vi "Wysyllanie danych do PC .vi"(5 "remote port":u16, 6 "output cluster 2":T2 {"CAN frame"."type" items=["CAN Data", "CAN Remote"]; "CAN frame"."identifier" format="%.0x"}, 7 "adres":u32, 8 "error in (no error)":errorcluster, 11 "UDP Network Connection in":refnum<k16>) -> (0 "error out":errorcluster, 3 "UDP Network Connection out":refnum<k16>)   [LabVIEW 2015]
uses:
  <vilib>/RioEmbeddedCAN/RioEmbeddedCAN.llb/CANFrameControl.ctl
panel:
  out "length":i32
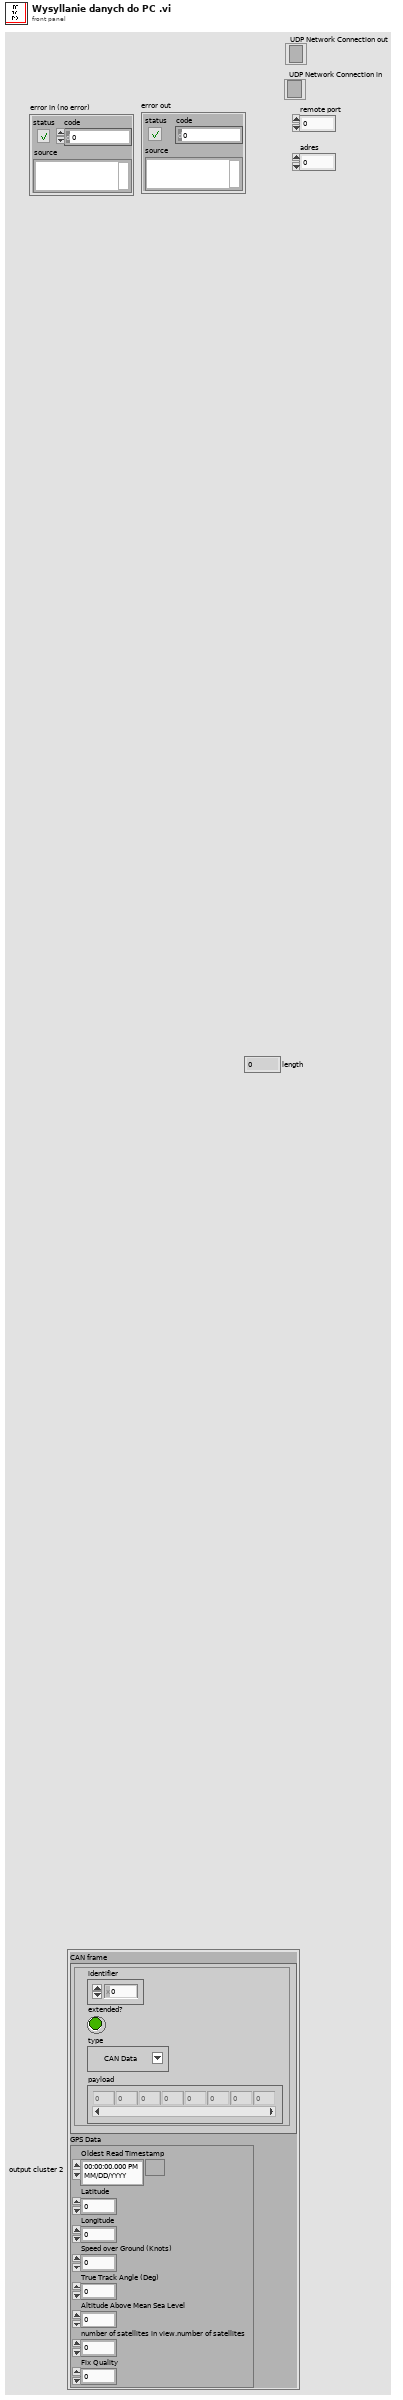
[diagram p1: front panel]
types:
  T1 = typedef "CANFrameControl.ctl" = cluster{"identifier":u32, "extended?":bool, "type":u8, "payload":u8[]}
  T2 = cluster{"CAN frame":T1, "GPS Data":cluster{"Oldest Read Timestamp":timestamp, "Latitude":dbl, "Longitude":dbl, "Speed over Ground (Knots)":dbl, "True Track Angle (Deg)":dbl, "Altitude Above Mean Sea Level":dbl, "number of satellites in view.number of satellites":i8, "Fix Quality ":u16}}
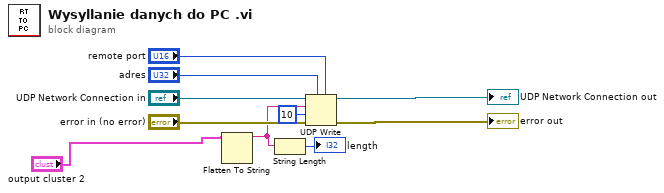
[diagram p0: block diagram]
diagram:
  n1 = Flatten To String(anything="output cluster 2") -> (data string=w3:string)  [unwired: 3 in, 2 out]
  n2 = String Length(string=w3) -> (length=→"length":i32)
  n3 = UDP Write(address="adres", port or service name="remote port", connection ID="UDP Network Connection in", data in=w3, 8:"error in (no error)", 9:10 ("timeout ms (25000)")) -> (error out=→"error out":errorcluster, 3:→"UDP Network Connection out":refnum<k16>)
